vi "Serialize - Text.vi"(8 "error in (no error)":errorcluster, 11 "mTEC Data in":refnum<class "mTEC Data.lvclass">) -> (0 "error out":errorcluster, 2 "Serialized Text":string, 3 "mTEC Data out":refnum<class "mTEC Data.lvclass">)   [LabVIEW 2014, in "Meerstetter Lib.lvlib" / "mTEC Data.lvclass"]
uses:
  mTEC Data.lvclass
  mTEC Data.lvclass/mTEC Data.ctl
  reusable/Data/Data.lvclass
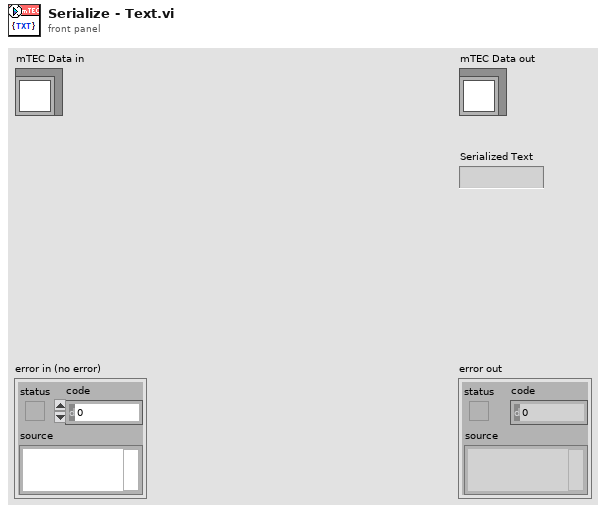
[diagram p1: front panel]
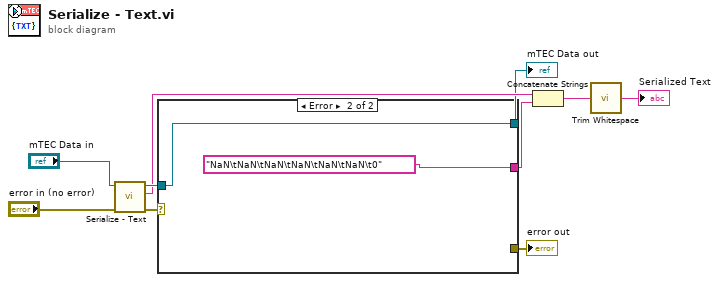
[diagram p0: block diagram]
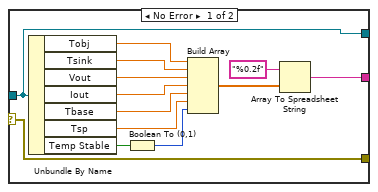
[diagram p2: hidden frame]
diagram:
  n1 = call-parent "Serialize - Text.vi"("error in"="error in (no error)", "Data in"="mTEC Data in") -> ("error out"=w3:errorcluster, "Serialized Text"=w6:string, "Data out"=w8:refnum<class "mTEC Data.lvclass">)  [unwired: 7 in]
  n2 = case shown="Error" w3 {
    selector: w3 -> [w11 _]
    tunnel: w8 -> [w12 w24]
    tunnel: [w13 "NaN\tNaN\tNaN\tNaN\tNaN\tNaN\t0"] -> w4
    tunnel: [w12 w24] -> w2
    tunnel: [w11 _] -> w1
    frame No Error {
      n3 = Unbundle By Name(w12) -> ("Tobj"=w23:dbl, "Tsink"=w22:dbl, "Vout"=w21:dbl, "Iout"=w17:dbl, "Tbase"=w16:dbl, "Tsp"=w15:dbl, "Temp Stable"=w18:bool)
      n4 = Boolean To (0,1)(Boolean=w18) -> (0, 1=w14:i16)
      n5 = Build Array(w23, w22, w21, w17, w16, w15, w14) -> (w20:dbl[])
      n6 = Array To Spreadsheet String(array=w20, 3:"%0.2f" ("format string")) -> (spreadsheet string=w13:string)  [unwired: 1 in]
    }
    frame Error {
    }
  }
  "error out" <- w1
  "mTEC Data out" <- w2
  n7 = Concatenate Strings(w6, w4) -> (w5:string)
  n8 = call <vilib>:"Trim Whitespace.vi"("string"=w5) -> ("trimmed string"=→"Serialized Text":string)  [unwired: 1 in]
